vi "Swerve Drive Published Globals.vi"() -> ()   [LabVIEW 2015]
panel:
  out "Rotation Angle Cluster":T1 {"FL Angle" scale=3.1416..-3.1416; "FR Angle" scale=3.1416..-3.1416; "RR Angle" scale=3.1416..-3.1416; "RL Angle" scale=3.1416..-3.1416}
  out "Rotation Multipliers":T2
  in  "Drive Train Absolute Offsets (ticks)":dbl[](array[numeric])=[-0.395, 1.11, 1.68, -1.896]
  in  "Wheel Angle Invert":bool
  in  "Absolute Encoder TPR":dbl
  in  "Robot Height":dbl=24.0
  in  "Robot Width":dbl=24.0
  # "Tip: The global is a good way publish state or\ninformational/debugging values.\nIt is not  advised that you put setpoint values here."
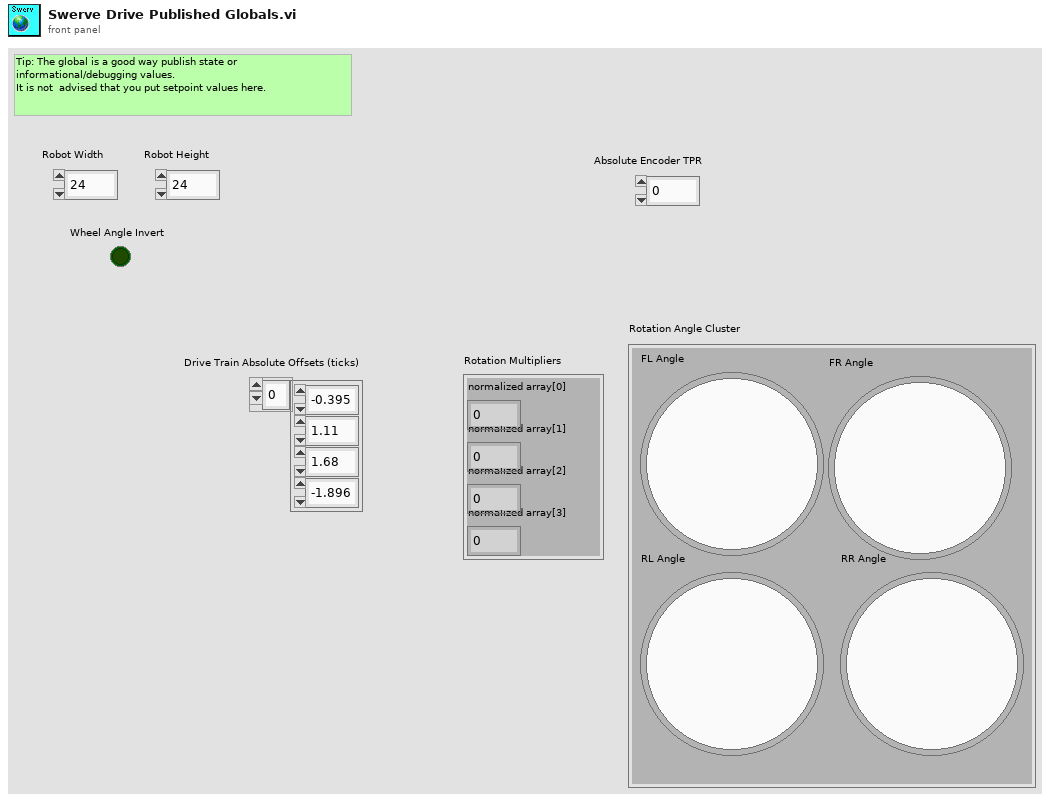
[diagram p1: front panel]
types:
  T1 = cluster{"FL Angle":dbl, "FR Angle":dbl, "RL Angle":dbl, "RR Angle":dbl}
  T2 = cluster{"normalized array[0]":dbl, "normalized array[1]":dbl, "normalized array[2]":dbl, "normalized array[3]":dbl}
diagram:
